vi "CenterWidth_to_StartEnd.vi"(10 "width":dbl, 11 "Center":dbl) -> (2 "Start":dbl, 3 "End":dbl)   [LabVIEW 2020]
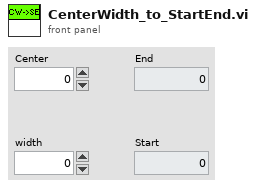
[diagram p1: front panel]
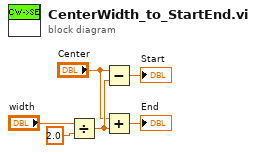
[diagram p0: block diagram]
diagram:
  n1 = Divide(x="width", y=2.0) -> (x/y=w4:dbl)
  n2 = Subtract(x="Center", y=w4) -> (x-y=→"Start":dbl)
  n3 = Add(x="Center", y=w4) -> (x+y=→"End":dbl)
